vi "GetFormat.vi"() -> (0 "NPdark":i32, 1 "NPtotal":i32=512, 2 "NSoverscan":i32, 3 "NSunderscan":i32, 4 "NPunderscan":i32, 5 "NSdark":i32, 6 "NPoverscan":i32, 7 "NStotal":i32=512, 8 "NPframetransfer":i32=512)   [LabVIEW 2014]
panel:
  out "Error":bool
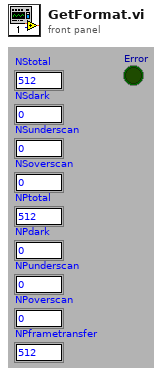
[diagram p1: front panel]
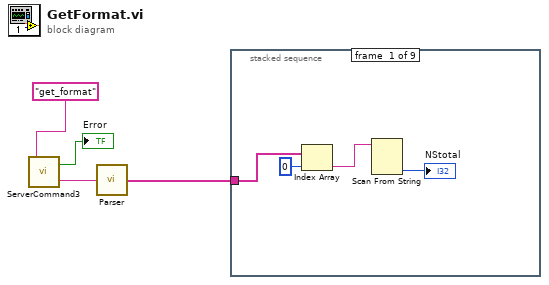
[diagram p0: block diagram]
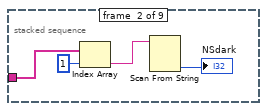
[diagram p2: hidden frame]
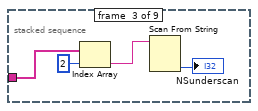
[diagram p3: hidden frame]
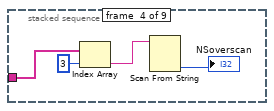
[diagram p4: hidden frame]
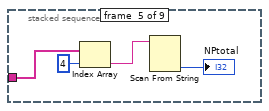
[diagram p5: hidden frame]
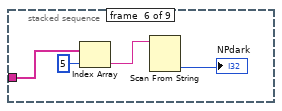
[diagram p6: hidden frame]
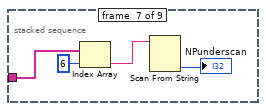
[diagram p7: hidden frame]
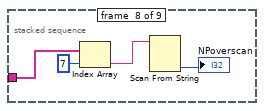
[diagram p8: hidden frame]
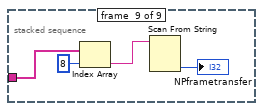
[diagram p9: hidden frame]
diagram:
  n1 = call "ServerCommand3.vi"("Command"="get_format") -> ("Error"=→"Error":bool, "Reply"=w3:string)
  n2 = call "Parser.vi"("string"=w3) -> ("Out Strings"=w1:string[])
  n3 = stacked-sequence {
    tunnel: w1 -> [w7 w12 w16 w20 w24 w28 w32 w36 w40]
    frame #0 {
      n4 = Index Array(array=w7, index=0) -> (element=w5:string)
      n5 = Scan From String(input string=w5) -> (output 1=→"NStotal":i32)  [unwired: 4 in, 3 out]
    }
    frame #1 {
      n6 = Index Array(array=w12, index=1) -> (element=w10:string)
      n7 = Scan From String(input string=w10) -> (output 1=→"NSdark":i32)  [unwired: 4 in, 3 out]
    }
    frame #2 {
      n8 = Index Array(array=w16, index=2) -> (element=w14:string)
      n9 = Scan From String(input string=w14) -> (output 1=→"NSunderscan":i32)  [unwired: 4 in, 3 out]
    }
    frame #3 {
      n10 = Index Array(array=w20, index=3) -> (element=w18:string)
      n11 = Scan From String(input string=w18) -> (output 1=→"NSoverscan":i32)  [unwired: 4 in, 3 out]
    }
    frame #4 {
      n12 = Index Array(array=w24, index=4) -> (element=w22:string)
      n13 = Scan From String(input string=w22) -> (output 1=→"NPtotal":i32)  [unwired: 4 in, 3 out]
    }
    frame #5 {
      n14 = Index Array(array=w28, index=5) -> (element=w26:string)
      n15 = Scan From String(input string=w26) -> (output 1=→"NPdark":i32)  [unwired: 4 in, 3 out]
    }
    frame #6 {
      n16 = Index Array(array=w32, index=6) -> (element=w30:string)
      n17 = Scan From String(input string=w30) -> (output 1=→"NPunderscan":i32)  [unwired: 4 in, 3 out]
    }
    frame #7 {
      n18 = Index Array(array=w36, index=7) -> (element=w34:string)
      n19 = Scan From String(input string=w34) -> (output 1=→"NPoverscan":i32)  [unwired: 4 in, 3 out]
    }
    frame #8 {
      n20 = Index Array(array=w40, index=8) -> (element=w38:string)
      n21 = Scan From String(input string=w38) -> (output 1=→"NPframetransfer":i32)  [unwired: 4 in, 3 out]
    }
  }
